vi "User_Defined_Test_PID.vi"() -> (3 "Unit Test Framework Results":T1)   [LabVIEW 2016]
doc: "Use this template to create a user-defined test VI. Define your test requirements and wire the results to the <b>Result (Test)</b> control. Do not modify the <b>Unit Test Framework Results</b> indicator."
uses:
  <vilib>/utf/common/utf_test_result_troll.ctl
  <vilib>/utf/common/utf_test_result.ctl
  <vilib>/utf/common/utf_test_result_failure.ctl
  <vilib>/utf/common/utf_test_comparison_operators.ctl
  <vilib>/utf/common/utf_vi_tag.ctl
  <vilib>/Control Software Solutions Ltd/UTF Helper/SubVIs/UTF Boolean Equals.vi
  <vilib>/Control Software Solutions Ltd/UTF Helper/SubVIs/UTF Double Equals.vi
  MyPAM Controller/controllerLibrary.lvlib
  <vilib>/Control Software Solutions Ltd/UTF Helper/Unit Test Helper.lvlib
  <vilib>/utf/NI_UnitTestFramework.lvlib
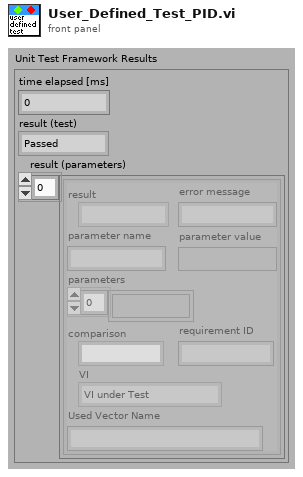
[diagram p1: front panel]
types:
  T1 = typedef "NI_UnitTestFramework.lvlib/utf_test_result_troll.ctl" = cluster{"time elapsed [ms]":u32, "result (test)":T2, "result (parameters)":T3[]}
  T2 = typedef "NI_UnitTestFramework.lvlib/utf_test_result.ctl" = enum16{"Passed", "Failed", "Error", "Skipped", "Not Processed"}
  T3 = typedef "NI_UnitTestFramework.lvlib/utf_test_result_failure.ctl" = cluster{"result":T2, "error message":string, "parameter name":string, "parameter value":variant, "parameters":variant[], "comparison":T4, "requirement ID":string, "VI":T5, "Used Vector Name":string}
  T4 = typedef "NI_UnitTestFramework.lvlib/utf_test_comparison_operators.ctl" = enum16{"=", "!=", ">", ">=", "<", "<=", "range", "symmetric tolerance", "asymmetric tolerance", "string contains", "string not contain", "array size", "string length", "array range", "by element", "array range (limit array)", "user-defined", "array contains", "array not contain", "vector length", "= (elm)", "!= (elm)", "= (case insensitive)", "!= (case insensitive)"}
  T5 = typedef "NI_UnitTestFramework.lvlib/utf_vi_tag.ctl" = enum16{"Setup VI", "VI under Test", "Teardown VI"}
  T6 = cluster{"proportional gain (Kc)":dbl, "integral time (Ti, min)":dbl, "derivative time (Td, min)":dbl}
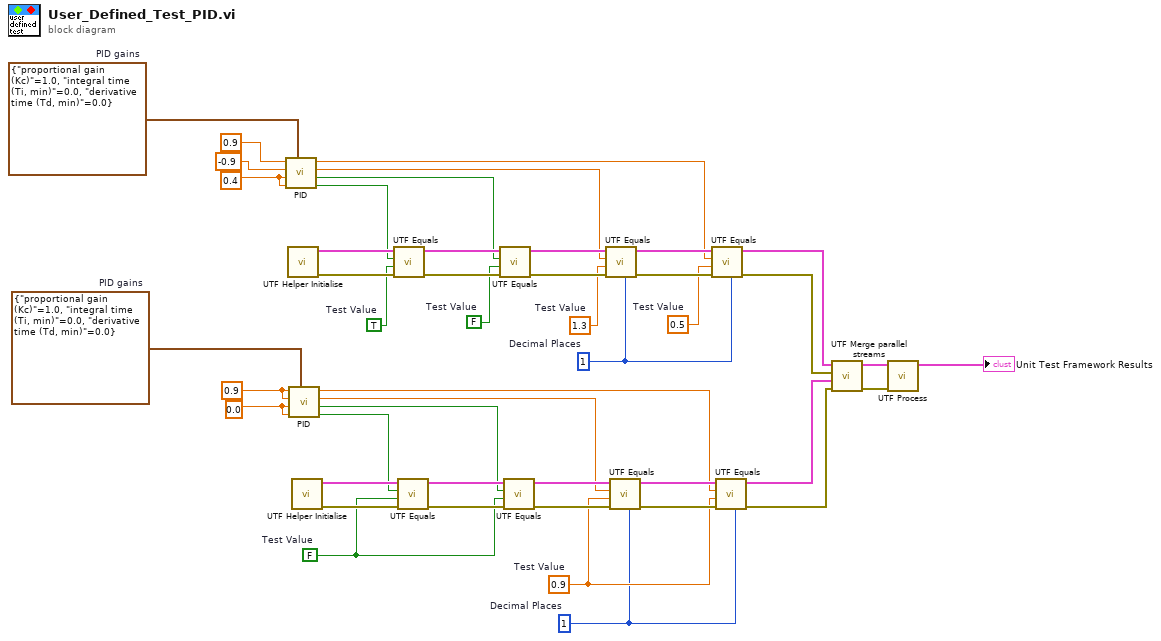
[diagram p0: block diagram]
diagram:
  w7 = u8 1  # Decimal Places
  w8 = u8 1  # Decimal Places
  w9 = 0.5  # Test Value
  w10 = 1.3  # Test Value
  w11 = TRUE  # Test Value
  w12 = FALSE  # Test Value
  w20 = 0.4 ("Des theta0")
  w19 = T6 {"proportional gain (Kc)"=1.0, "integral time (Ti, min)"=0.0, "derivative time (Td, min)"=0.0}  # PID gains
  w21 = 0.9  # Test Value
  w22 = FALSE  # Test Value
  w27 = 0.0 ("Des theta0")
  w28 = 0.9 ("Des theta0")
  w29 = T6 {"proportional gain (Kc)"=1.0, "integral time (Ti, min)"=0.0, "derivative time (Td, min)"=0.0}  # PID gains
  n1 = call "PID.vi"("PID gains"=w19, "current theta1"=w20, "current theta0"=w20, "Des theta1"=-0.9 ("Des theta0"), "Des theta0"=0.9) -> ("Dir2"=w13:bool, "Dir1"=w14:bool, "U2"=w15:dbl, "U1"=w16:dbl)  [unwired: 3 in]
  n2 = call <vilib>:"UTF Helper Initialise.vi"() -> ("error out"=w31:errorcluster, "results array"=w30:T3[])  [unwired: 10 in]
  n3 = call "PID.vi"("PID gains"=w29, "current theta1"=w27, "current theta0"=w27, "Des theta1"=w28, "Des theta0"=w28) -> ("Dir2"=w23:bool, "Dir1"=w24:bool, "U2"=w25:dbl, "U1"=w26:dbl)  [unwired: 3 in]
  n4 = call <vilib>:"UTF Helper Initialise.vi"() -> ("error out"=w44:errorcluster, "results array"=w45:T3[])  [unwired: 10 in]
  n5 = call-poly <vilib>:"UTF Equals.vi"("error in (no error)"=w31, "Test Value"=w11, "Input"=w13, "Input Results"=w30) -> ("error out"=w33:errorcluster, "Output Results"=w32:T3[])  [unwired: 6 in]
  n6 = call-poly <vilib>:"UTF Equals.vi"("error in (no error)"=w44, "Test Value"=w22, "Input"=w23, "Input Results"=w45) -> ("error out"=w42:errorcluster, "Output Results"=w43:T3[])  [unwired: 6 in]
  n7 = call-poly <vilib>:"UTF Equals.vi"("error in (no error)"=w33, "Test Value"=w12, "Input"=w14, "Input Results"=w32) -> ("error out"=w35:errorcluster, "Output Results"=w34:T3[])  [unwired: 6 in]
  n8 = call-poly <vilib>:"UTF Equals.vi"("error in (no error)"=w42, "Test Value"=w22, "Input"=w24, "Input Results"=w43) -> ("error out"=w40:errorcluster, "Output Results"=w41:T3[])  [unwired: 6 in]
  n9 = call-poly <vilib>:"UTF Equals.vi"("Decimal Places"=w8, "error in (no error)"=w35, "Test Value"=w10, "Input"=w15, "Input Results"=w34) -> ("error out"=w37:errorcluster, "Output Results"=w36:T3[])  [unwired: 5 in]
  n10 = call-poly <vilib>:"UTF Equals.vi"("Decimal Places"=w7, "error in (no error)"=w40, "Test Value"=w21, "Input"=w25, "Input Results"=w41) -> ("error out"=w38:errorcluster, "Output Results"=w39:T3[])  [unwired: 5 in]
  n11 = call-poly <vilib>:"UTF Equals.vi"("Decimal Places"=w8, "error in (no error)"=w37, "Test Value"=w9, "Input"=w16, "Input Results"=w36) -> ("error out"=w5:errorcluster, "Output Results"=w6:T3[])  [unwired: 5 in]
  n12 = call-poly <vilib>:"UTF Equals.vi"("Decimal Places"=w7, "error in (no error)"=w38, "Test Value"=w21, "Input"=w26, "Input Results"=w39) -> ("error out"=w3:errorcluster, "Output Results"=w4:T3[])  [unwired: 5 in]
  n13 = call <vilib>:"UTF Merge parallel streams.vi"("error in 2"=w3, "Results input 2"=w4, "error in 1"=w5, "Results input 1"=w6) -> ("error out"=w1:errorcluster, "Concatenated Results"=w2:T3[])  [unwired: 6 in]
  n14 = call <vilib>:"UTF Process.vi"("error in (no error)"=w1, "results array"=w2) -> ("Unit Test Framework Results"=→"Unit Test Framework Results":T1)  [unwired: 9 in]
